vi "Set Save Settings.vi"(7 "Remove block diagram (false)":bool, 8 "error in (no error)":errorcluster, 9 "Remove front panel (false)":bool, 10 "ProjectItem Refnum":refnum<vi>, 11 "SDIST in":refnum<class "NI_AB_API_SDIST.lvclass">) -> (0 "error out":errorcluster, 3 "SDIST out":refnum<class "NI_AB_API_SDIST.lvclass">)   [LabVIEW 2020, in "NI_AB_API_SDIST.lvclass"]
uses:
  <vilib>/AppBuilder/AB_API/SDIST/NI_AB_API_SDIST.lvclass
  e:/builds/penguin/labview/branches/2020/dev/dist/vi.lib/AppBuilder/AB_API/Build/NI_AB_API_Build.lvclass
  <vilib>/AppBuilder/AB_Classes/SourceDistribution/AB_SourceDistribution.lvclass
  e:/builds/penguin/labview/branches/2020/dev/dist/vi.lib/AppBuilder/AB_Classes/Build/AB_Build.lvclass
  <vilib>/AppBuilder/AB_Classes/Build/AB_Build.lvclass
  <vilib>/AppBuilder/AB_API/Build/NI_AB_API_Build.lvclass
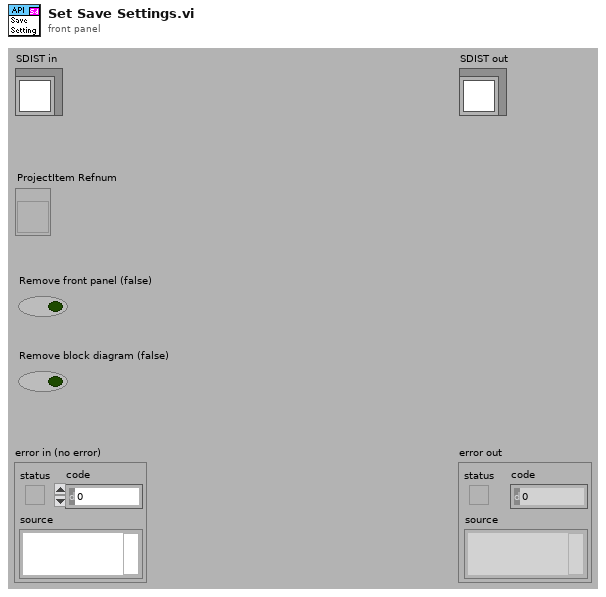
[diagram p1: front panel]
types:
  T1 = typedef "AB_Build.ctl" = cluster{"buildSpecName":string, "buildSpecDescription":string, "destinations":refnum<class "AB_Destination.lvclass">[], "exclusionOption":T2, "defaultLanguage":string, "supportedLanguages":string[], "excludedDirectories":path[], "buildContext":refnum<vi>, "buildObject":T3, "preview":bool, "programatic":bool, "progressBarEvents":T4, "userLog_Path":path, "preActionID":string, "preAction_Path":path, "postActionID":string, "postAction_Path":path, "eng_checkForBrokenVIs?":bool, "eng_verboseLinkerErrors?":bool, "localDest_Path":path, "targetDest_Path":path, "removeVIObject":u16, "cache":refnum<class "PreviewCache.lvclass">, "use cache":bool, "previewCache_ID":string, "buildCache_ID":string, "eng_TempLocalDest_Path":path, "eng_collectDependencies?":bool, "versionInfo":cluster{"buildVersion":cluster{"major":u16, "minor":u16, "patch":u16, "build":u16}, "autoIncrement":bool}, "eng_enableVIChecksums":bool}
  T2 = typedef "AB_Exclusion_Option.ctl" = cluster{"typedefs":bool, "polymorphicVIs":bool, "unusedLibraryItems":bool, "modifyLibraryFile":bool, "edit-timeDependencies":bool, "inlineVIs":bool, "dependent PPLs":bool, "dependent DLLs":bool}
  T3 = typedef "ItemRef.ctl" = u64
  T4 = typedef "provcom_ProgressBar_Events.ctl" = cluster{"newJob":refnum<user-event>, "newItem":refnum<user-event>, "errorMsg":T5, "cancel":refnum<user-event>}
  T5 = typedef "mxLvBuildError.ctl" = refnum<user-event>
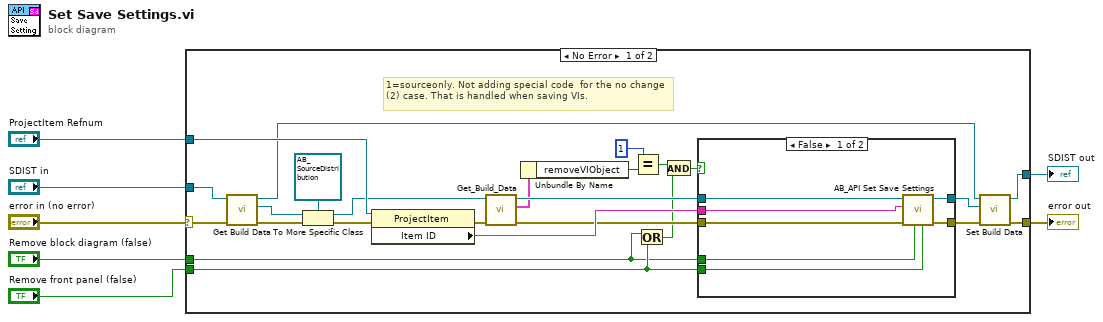
[diagram p0: block diagram]
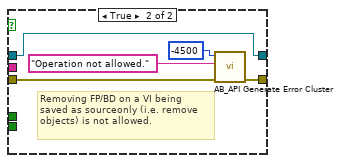
[diagram p2: hidden frame]
diagram:
  n1 = case shown="No Error" "error in (no error)" {
    selector: "error in (no error)" -> [w16 w46]
    tunnel: [w21 w46] -> w6
    tunnel: [w19 w45] -> w4
    tunnel: "SDIST in" -> [w25 w45]
    tunnel: "ProjectItem Refnum" -> [w32 _]
    tunnel: "Remove block diagram (false)" -> [w8 _]
    tunnel: "Remove front panel (false)" -> [w9 _]
    frame No Error {
      # "1=sourceonly. Not adding special code  for the no change (2) case. That is handled when saving VIs."
      n2 = call <vilib>:"Get Build Data.vi"("error in (no error)"=w16, "NI_AB_API_Build in"=w25) -> ("error out"=w14:errorcluster, "AB_Build.lvclass"=w24:refnum<class "AB_Build.lvclass">, "NI_AB_API_Build out"=w18:refnum<class "NI_AB_API_SDIST.lvclass">)  [unwired: 7 in]
      n3 = To More Specific Class(target class=refnum<class "AB_SourceDistribution.lvclass"> refnum ("AB_SourceDistribution.lvclass"), reference=w24, error in=w14) -> (specific class reference=w23:refnum<class "AB_SourceDistribution.lvclass">, error out=w13:errorcluster)
      n4 = property class="ProjectItem"(reference=w32, error in=w13) -> (error out=w15:errorcluster, "Item ID"=w31:string)  [unwired: 1 out]
      n5 = call <vilib>:"Get_Build_Data.vi"("error in (no error)"=w15, "Class in"=w23) -> ("error out"=w29:errorcluster, "data"=w28:T1, "Class out"=w30:refnum<class "AB_SourceDistribution.lvclass">)  [unwired: 7 in]
      n6 = Unbundle By Name(w28) -> ("removeVIObject"=w12:u16)
      n7 = Equal?(x=u16 1, y=w12) -> (x = y?=w10:bool)
      n8 = Or(x=w8, y=w9) -> (x .or. y?=w27:bool)
      n9 = And(x=w10, y=w27) -> (x .and. y?=w26:bool)
      n10 = case shown="False" w26 {
        tunnel: [w39 w44] -> w17
        tunnel: w31 -> [w38 _]
        tunnel: [w37 w41] -> w20
        tunnel: w30 -> [w36 w44]
        tunnel: w29 -> [w35 w40]
        tunnel: w8 -> [w34 _]
        tunnel: w9 -> [w33 _]
        frame False {
          n11 = call <vilib>:"AB_API Set Save Settings.vi"("Remove front panel (false)"=w33, "Remove block diagram (false)"=w34, "error in (no error)"=w35, "source item ID"=w38, "Build in"=w36) -> ("error out"=w37:errorcluster, "Build out"=w39:refnum<class "AB_SourceDistribution.lvclass">)  [unwired: 5 in]
        }
        frame True {
          # "Removing FP/BD on a VI being saved as sourceonly (i.e. remove objects) is not allowed."
          n12 = call <vilib>:"AB_API Generate Error Cluster.vi"("error in (no error)"=w40, "Additional Message"="Operation not allowed.", "Code"=-4500) -> ("error out"=w41:errorcluster)  [unwired: 1 in, 7 out]
        }
      }
      n13 = call <vilib>:"Set Build Data.vi"("error in (no error)"=w20, "AB_Build.lvclass"=w17, "NI_AB_API_Build in"=w18) -> ("error out"=w21:errorcluster, "NI_AB_API_Build out"=w19:refnum<class "NI_AB_API_SDIST.lvclass">)  [unwired: 7 in]
    }
    frame Error {
    }
  }
  "error out" <- w6
  "SDIST out" <- w4
